vi "GenerateSequence.vi"(8 "error in (no error)":errorcluster, 11 "SequenceIndices":refnum<class "SequenceIndex.lvclass">[](array[class])) -> (0 "error out":errorcluster, 3 "SequenceIndexValues":refnum<class "VariableValue.lvclass">[][](array[class]))   [LabVIEW 2013, in "VariableManager.lvclass"]
doc: "Generate sequence indices values for variable evaluation."
uses:
  VariableManager.lvclass
  VariableValue/VariableValue.lvclass
  SequenceIndex/SequenceIndex.lvclass
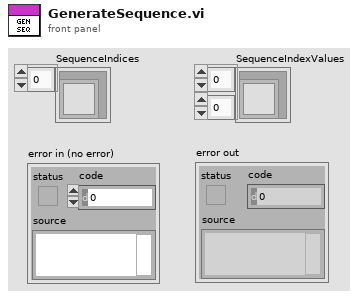
[diagram p1: front panel]
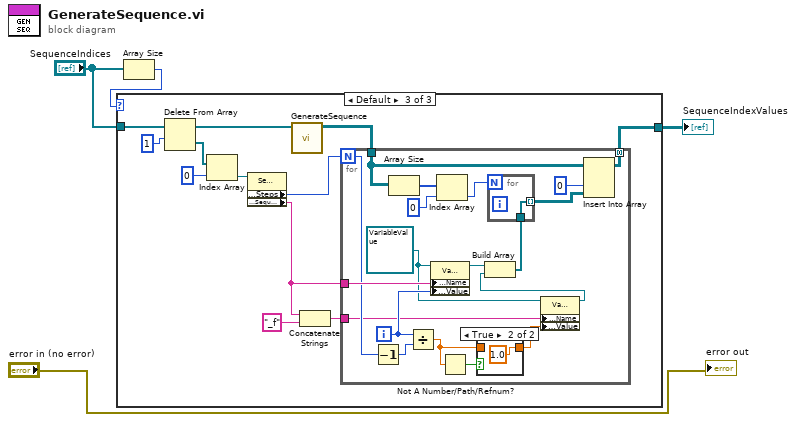
[diagram p0: block diagram]
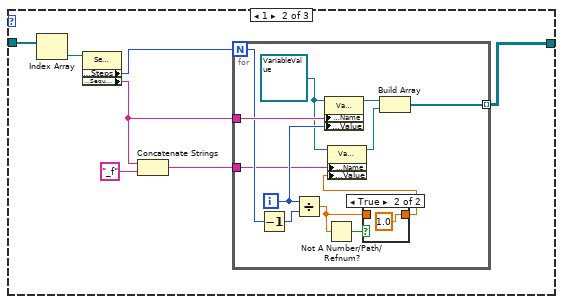
[diagram p3: hidden frame]
diagram:
  n1 = Array Size(array="SequenceIndices") -> (size(s)=w3:i32)
  n2 = case shown="Default" w3 {
    tunnel: "SequenceIndices" -> [_ w11 w37]
    tunnel: [_ w8 w32] -> w4
    frame 0 {
    }
    frame 1 {
      n3 = Index Array(array=w11) -> (element=w10:refnum<class "SequenceIndex.lvclass">)  [unwired: 1 in]
      n4 = property class="SequenceIndex.lvclass"(reference=w10) -> ("Accessors:Steps"=w9:u32, "Accessors:SequenceIndexName"=w7:string)  [unwired: 1 in, 2 out]
      n5 = Concatenate Strings(w7, "_f") -> (w5:string)
      n6 = for {
        N: w9 -> [w17]
        tunnel: w7 -> [w22]
        tunnel: [w23] -> w8 mode=indexing
        tunnel: w5 -> [w13]
        i -> [w16]
        w15 = refnum<class "VariableValue.lvclass"> refnum ("VariableValue.lvclass")
        n7 = Decrement(x=w17) -> (x-1=w18:i32)
        n8 = Divide(x=w16, y=w18) -> (x/y=w20:dbl)
        n9 = property class="VariableValue.lvclass"(reference=w15, "Accessors:Name"=w22, "Accessors:Value"=w16) -> (reference out=w21:refnum<class "VariableValue.lvclass">)  [unwired: 1 in, 1 out]
        n10 = Not A Number/Path/Refnum?(number/path/refnum=w20) -> (NaN/Path/Refnum?=w19:bool)
        n11 = case shown="True" w19 {
          tunnel: w20 -> [w24 _]
          tunnel: [w24 1.0] -> w12
          frame False {
          }
          frame True {
          }
        }
        n12 = property class="VariableValue.lvclass"(reference=w15, "Accessors:Name"=w13, "Accessors:Value"=w12) -> (reference out=w14:refnum<class "VariableValue.lvclass">)  [unwired: 1 in, 1 out]
        n13 = Build Array(w21, w14) -> (w23:refnum<class "VariableValue.lvclass">[])
      }
    }
    frame Default {
      n14 = Delete From Array(array=w37, length=1) -> (deleted portion=w35:refnum<class "SequenceIndex.lvclass">[], array with subset deleted=w27:refnum<class "SequenceIndex.lvclass">[])  [unwired: 1 in]
      n15 = Index Array(array=w35, index=0) -> (element=w34:refnum<class "SequenceIndex.lvclass">)
      n16 = property class="SequenceIndex.lvclass"(reference=w34) -> ("Accessors:Steps"=w33:u32, "Accessors:SequenceIndexName"=w30:string)  [unwired: 1 in, 2 out]
      n17 = call "GenerateSequence.vi"("SequenceIndices"=w27) -> ("SequenceIndexValues"=w26:refnum<class "VariableValue.lvclass">[][])  [unwired: 9 in, 1 out]
      n18 = Concatenate Strings(w30, "_f") -> (w28:string)
      n19 = for {
        N: w33 -> [w46]
        tunnel: w30 -> [w49]
        tunnel: [w47] -> w32 mode=concatenating
        tunnel: w26 -> [w50]
        tunnel: w28 -> [w40]
        i -> [w45]
        w41 = refnum<class "VariableValue.lvclass"> refnum ("VariableValue.lvclass")
        n20 = Decrement(x=w46) -> (x-1=w44:i32)
        n21 = Array Size(array=w50) -> (size(s)=w55:i32[])
        n22 = Divide(x=w45, y=w44) -> (x/y=w42:dbl)
        n23 = property class="VariableValue.lvclass"(reference=w41, "Accessors:Name"=w49, "Accessors:Value"=w45) -> (reference out=w48:refnum<class "VariableValue.lvclass">)  [unwired: 1 in, 1 out]
        n24 = Index Array(array=w55, index=0) -> (element=w54:i32)
        n25 = Not A Number/Path/Refnum?(number/path/refnum=w42) -> (NaN/Path/Refnum?=w43:bool)
        n26 = case shown="True" w43 {
          tunnel: w42 -> [w57 _]
          tunnel: [w57 1.0] -> w39
          frame False {
          }
          frame True {
          }
        }
        n27 = property class="VariableValue.lvclass"(reference=w41, "Accessors:Name"=w40, "Accessors:Value"=w39) -> (reference out=w38:refnum<class "VariableValue.lvclass">)  [unwired: 1 in, 1 out]
        n28 = Build Array(w48, w38) -> (w53:refnum<class "VariableValue.lvclass">[])
        n29 = for {
          N: w54 -> [_]
          tunnel: w53 -> [w59]
          tunnel: [w59] -> w52 mode=indexing
        }
        n30 = Insert Into Array(array=w50, index (col)=0 ("disabled index (row)"), new element=w52) -> (w47:refnum<class "VariableValue.lvclass">[][])  [unwired: 1 in]
      }
    }
  }
  "SequenceIndexValues" <- w4
  "error out" <- "error in (no error)"
